vi "Bundle PXIe By Slot.vi"(11 "Analysis Info cluster":T1[](array[typedef]) {"Kurt_u" format="%_3g"; "u^4" format="%_3g"; "u^3" format="%_3g"; "Sd Error in Variance" format="%_3g"; "u^2" format="%_3g"; "Sd Error in Mean" format="%_3g"; "U" format="%_3g"; "Sync Delay Time (s)" format="%.4f"; "Total Meas Time (s)" format="%_5g"; "Skew_u" format="%_3g"; "% u'/U" format="%_3g"}) -> (2 "Slot 18":cluster{"Array":T1[]} {"Array"."Kurt_u" format="%_3g"; "Array"."u^4" format="%_3g"; "Array"."u^3" format="%_3g"; "Array"."Sd Error in Variance" format="%_3g"; "Array"."u^2" format="%_3g"; "Array"."Sd Error in Mean" format="%_3g"; "Array"."U" format="%_3g"; "Array"."Sync Delay Time (s)" format="%.4f"; "Array"."Total Meas Time (s)" format="%_5g"; "Array"."Skew_u" format="%_3g"; "Array"."% u'/U" format="%_3g"}, 3 "SG Slots":cluster{"Array":T1[]}[](array[cluster]) {"Array"."Kurt_u" format="%_3g"; "Array"."u^4" format="%_3g"; "Array"."u^3" format="%_3g"; "Array"."Sd Error in Variance" format="%_3g"; "Array"."u^2" format="%_3g"; "Array"."Sd Error in Mean" format="%_3g"; "Array"."U" format="%_3g"; "Array"."Sync Delay Time (s)" format="%.4f"; "Array"."Total Meas Time (s)" format="%_5g"; "Array"."Skew_u" format="%_3g"; "Array"."% u'/U" format="%_3g"}, 5 "All Slots":cluster{"Array":T1[]}[](array[cluster]) {"Array"."Kurt_u" format="%_3g"; "Array"."u^4" format="%_3g"; "Array"."u^3" format="%_3g"; "Array"."Sd Error in Variance" format="%_3g"; "Array"."u^2" format="%_3g"; "Array"."Sd Error in Mean" format="%_3g"; "Array"."U" format="%_3g"; "Array"."Sync Delay Time (s)" format="%.4f"; "Array"."Total Meas Time (s)" format="%_5g"; "Array"."Skew_u" format="%_3g"; "Array"."% u'/U" format="%_3g"})   [LabVIEW 2022 SP3]
uses:
  Controls/Analysis_info_cluster.ctl
  Controls/Inst_type.ctl
  Controls/Instrument_Array.ctl
  Controls/channelState.ctl
  64b3be66-aa39-4d9c-89d4-f8eecf134f84.vi
  daf71438-e10e-43e9-b3a7-33c3f8672ea4.vi
  Globals/Meas_global.vi
  <vilib>/Comparison/Less/Less Functor/Less Functor.lvclass
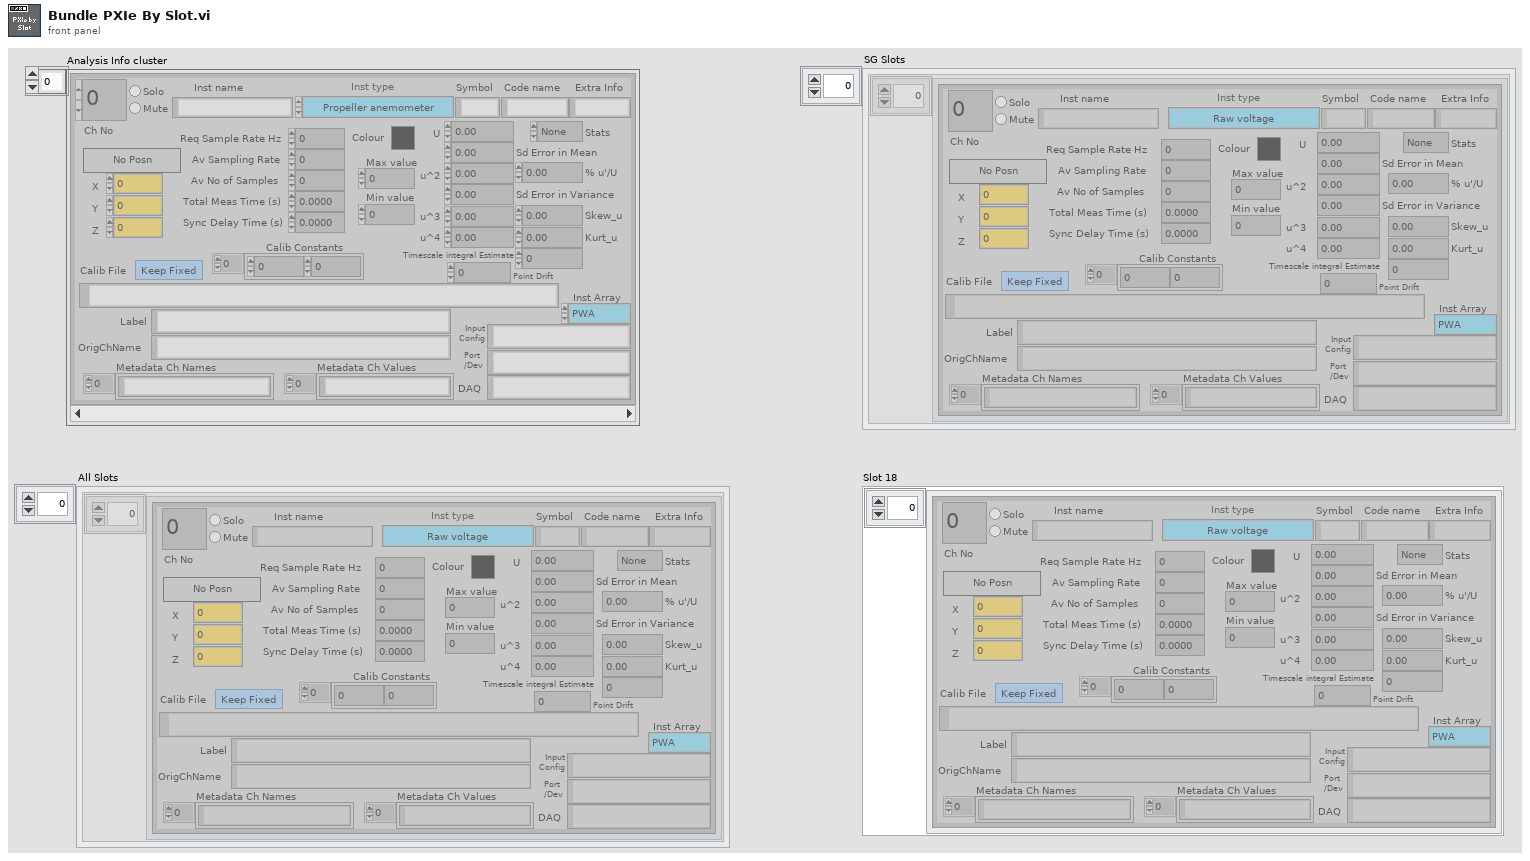
[diagram p1: front panel]
types:
  T1 = typedef "Analysis_info_cluster.ctl" = cluster{"Colour":u32, "Inst type":T2, "Inst name":string, "Symbol":string, "Code name":string, "Extra Info":string, "Inst Array":T3, "U":dbl, "u^2":dbl, "u^3":dbl, "u^4":dbl, "Skew_u":dbl, "Kurt_u":dbl, "Sd Error in Mean":dbl, "% u'/U":dbl, "X":dbl, "Y":dbl, "Z":dbl, "Timescale integral Estimate":dbl, "Sd Error in Variance":dbl, "Calib File":path, "Calib Constants":dbl[], "Output Position":bool, "Stats":enum16{"None", "Basic", "Full"}, "Av Sampling Rate":dbl, "Av No of Samples":dbl, "Total Meas Time (s)":dbl, "OrigChName":string, "Max value":dbl, "Min value":dbl, "Req Sample Rate Hz":dbl, "Sync Delay Time (s)":dbl, "Ch No":i16, "Device":string, "Use Latest Calib":bool, "Port":string, "Metadata Ch Names":string[], "Metadata Ch Values":string[], "Label":string, "chState":T4, "Point Drift":dbl, "inputConfig":string}
  T2 = typedef "Inst_type.ctl" = enum16{"Raw voltage", "Raw with zero offsetting", "Propeller anemometer", "Pressure Transducer", "Pitot-static tube", "Hot wire", "Cross wire 1", "Cross wire 2", "Generic Linear", "Generic Polynomial", "Generic BackPoly", "Fast FID", "Thermocouple", "Cold wire", "Pulsed Wire", "LDA Vel", "LDA Tran time", "LDA Arr time", "Microphone"}
  T3 = typedef "Instrument_Array.ctl" = enum16{"PWA", "LDA", "Analogue"}
  T4 = typedef "channelState.ctl" = enum32{"No Selection", "Solo", "Mute"}
  T5 = typedef "Rendezvous RefNum" = refnum<k1>
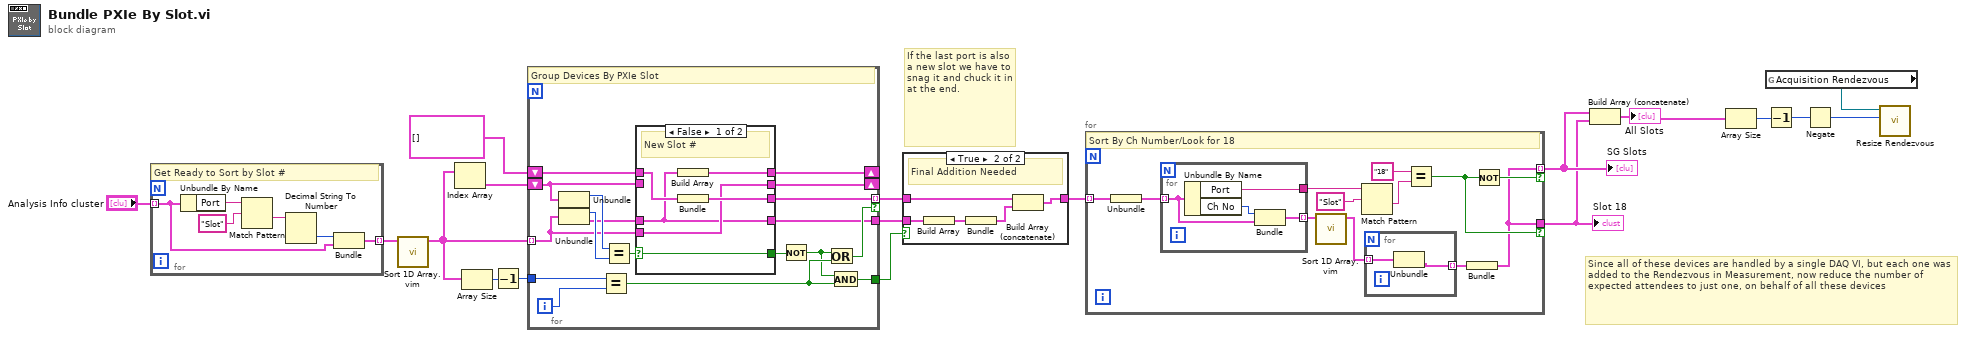
[diagram p0: block diagram]
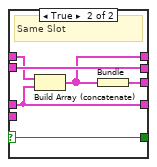
[diagram p3: hidden frame]
diagram:
  # "Since all of these devices are handled by a single DAQ VI, but each one was  added to the Rendezvous in Measurement, now reduce the number of expected attendees to just one, on behalf of all these devices"
  # "If the last port is also a new slot we have to snag it and chuck it in at the end."
  n1 = for {
    tunnel: "Analysis Info cluster" -> [w20] mode=indexing
    tunnel: [w19] -> w14 mode=indexing
    # "Get Ready to Sort by Slot #"
    n2 = Unbundle By Name(w20) -> ("Port"=w24:string)
    n3 = Match Pattern(string=w24, regular expression="Slot") -> (after substring=w22:string)  [unwired: 1 in, 3 out]
    n4 = Decimal String To Number(string=w22) -> (number=w21:i32)  [unwired: 2 in, 1 out]
    n5 = Bundle(w21, w20) -> (w19:cluster{i32, T1})  [unwired: 1 in]
  }
  n6 = call "Sort 1D Array.vim"("unsorted array"=w14) -> ("sorted array"=w13:cluster{i32, T1}[])  [unwired: 10 in]
  n7 = Index Array(array=w13) -> (element=w16:cluster{i32, T1})  [unwired: 1 in]
  n8 = Array Size(array=w13) -> (size(s)=w17:i32)
  n9 = Decrement(x=w17) -> (x-1=w18:i32)
  n10 = for {
    tunnel: w13 -> [w39] mode=indexing
    shift-right: [w37] -> _
    shift-left: w16 -> [w38]
    shift-right: [w36] -> _
    shift-left: T1[] [] -> [w31]
    tunnel: w18 -> [w35]
    tunnel: [w33] -> w10 mode=indexing if=w30
    tunnel: [w27] -> w11
    tunnel: [w25] -> w9
    i -> [w34]
    # "Group Devices By PXIe Slot"
    n11 = Unbundle(w38) -> (w42:i32)  [unwired: 1 out]
    n12 = Unbundle(w39) -> (w41:i32, w32:T1)
    n13 = Equal?(x=w35, y=w34) -> (x = y?=w28:bool)
    n14 = Equal?(x=w42, y=w41) -> (x = y?=w40:bool)
    n15 = case shown="False" w40 {
      selector: w40 -> [w45 w53]
      tunnel: w39 -> [w44 _]
      tunnel: w31 -> [w47 w50]
      tunnel: w38 -> [_ w54]
      tunnel: [w44 w54] -> w37
      tunnel: [w45 w53] -> w29
      tunnel: [w48 w52] -> w36
      tunnel: [w46 w51] -> w33
      tunnel: w32 -> [w43 w49]
      tunnel: [w43 w49] -> w25
      frame False {
        # "New Slot #"
        n16 = Build Array(w43) -> (w48:T1[])
        n17 = Bundle(w47) -> (w46:cluster{T1[]})  [unwired: 1 in]
      }
      frame True {
        # "Same Slot"
        n18 = Build Array (concatenate)(w50, w49) -> (w52:T1[])
        n19 = Bundle(w52) -> (w51:cluster{T1[]})  [unwired: 1 in]
      }
    }
    n20 = Not(x=w29) -> (.not. x?=w26:bool)
    n21 = Or(x=w26, y=w28) -> (x .or. y?=w30:bool)
    n22 = And(x=w26, y=w28) -> (x .and. y?=w27:bool)
  }
  n23 = case shown="True" w11 {
    tunnel: w10 -> [w55 w58]
    tunnel: w9 -> [_ w60]
    tunnel: [w55 w56] -> w8
    frame False {
      # "No Final Addition Needed"
    }
    frame True {
      # "Final Addition Needed"
      n24 = Build Array(w60) -> (w59:T1[])
      n25 = Bundle(w59) -> (w57:cluster{T1[]})  [unwired: 1 in]
      n26 = Build Array (concatenate)(w58, w57) -> (w56:cluster{T1[]}[])
    }
  }
  n27 = for {
    tunnel: w8 -> [w72] mode=indexing
    tunnel: [w61] -> w6 if=w64
    tunnel: [w61] -> w7 mode=indexing if=w65
    # "Sort By Ch Number/Look for 18"
    n28 = Unbundle(w72) -> (w71:T1[])
    n29 = for {
      tunnel: w71 -> [w77] mode=indexing
      tunnel: [w76] -> w70 mode=indexing
      tunnel: [w75] -> w68
      n30 = Unbundle By Name(w77) -> ("Port"=w75:string, "Ch No"=w78:i16)
      n31 = Bundle("Ch No"=w78, w77) -> (w76:cluster{"Ch No":i16, T1})  [unwired: 1 in]
    }
    n32 = call "Sort 1D Array.vim"("unsorted array"=w70) -> ("sorted array"=w63:cluster{"Ch No":i16, T1}[])  [unwired: 10 in]
    n33 = Match Pattern(string=w68, regular expression="Slot") -> (after substring=w66:string)  [unwired: 1 in, 3 out]
    n34 = for {
      tunnel: w63 -> [w74] mode=indexing
      tunnel: [w73] -> w62 mode=indexing
      n35 = Unbundle(w74) -> (w73:T1)  [unwired: 1 out]
    }
    n36 = Equal?(x="18" ("regular expression"), y=w66) -> (x = y?=w64:bool)
    n37 = Bundle(w62) -> (w61:cluster{T1[]})  [unwired: 1 in]
    n38 = Not(x=w64) -> (.not. x?=w65:bool)
  }
  "SG Slots" <- w7
  "Slot 18" <- w6
  n39 = Build Array (concatenate)(w7, w6) -> (w4:cluster{T1[]}[])
  "All Slots" <- w4
  n40 = Array Size(array=w4) -> (size(s)=w3:i32)
  n41 = global read "Meas_global.vi" "Acquisition Rendezvous"() -> (w5:T5)
  n42 = Decrement(x=w3) -> (x-1=w2:i32)
  n43 = Negate(x=w2) -> (-x=w1:i32)
  n44 = call <vilib>:"Resize Rendezvous.vi"("size change (0)"=w1, "rendezvous"=w5) -> ()  [unwired: 3 in, 3 out]
